vi "update devices in UI.vi"() -> ()   [LabVIEW 2025]
uses:
  <resource>/objmgr/niflexrioatomicsae.rc
panel:
  out "Ring Text.Text":string
  in  "Text Ring":u16(ring) items=["PXI1Slot2", "PXI1Slot5"]
  out "Array":string[](array[string])
  out "ProdName":string
  out "Found":bool
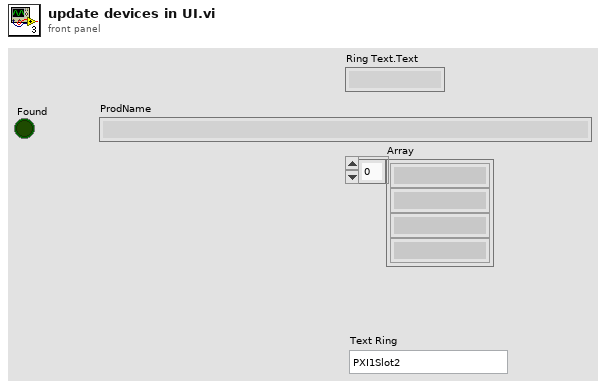
[diagram p1: front panel]
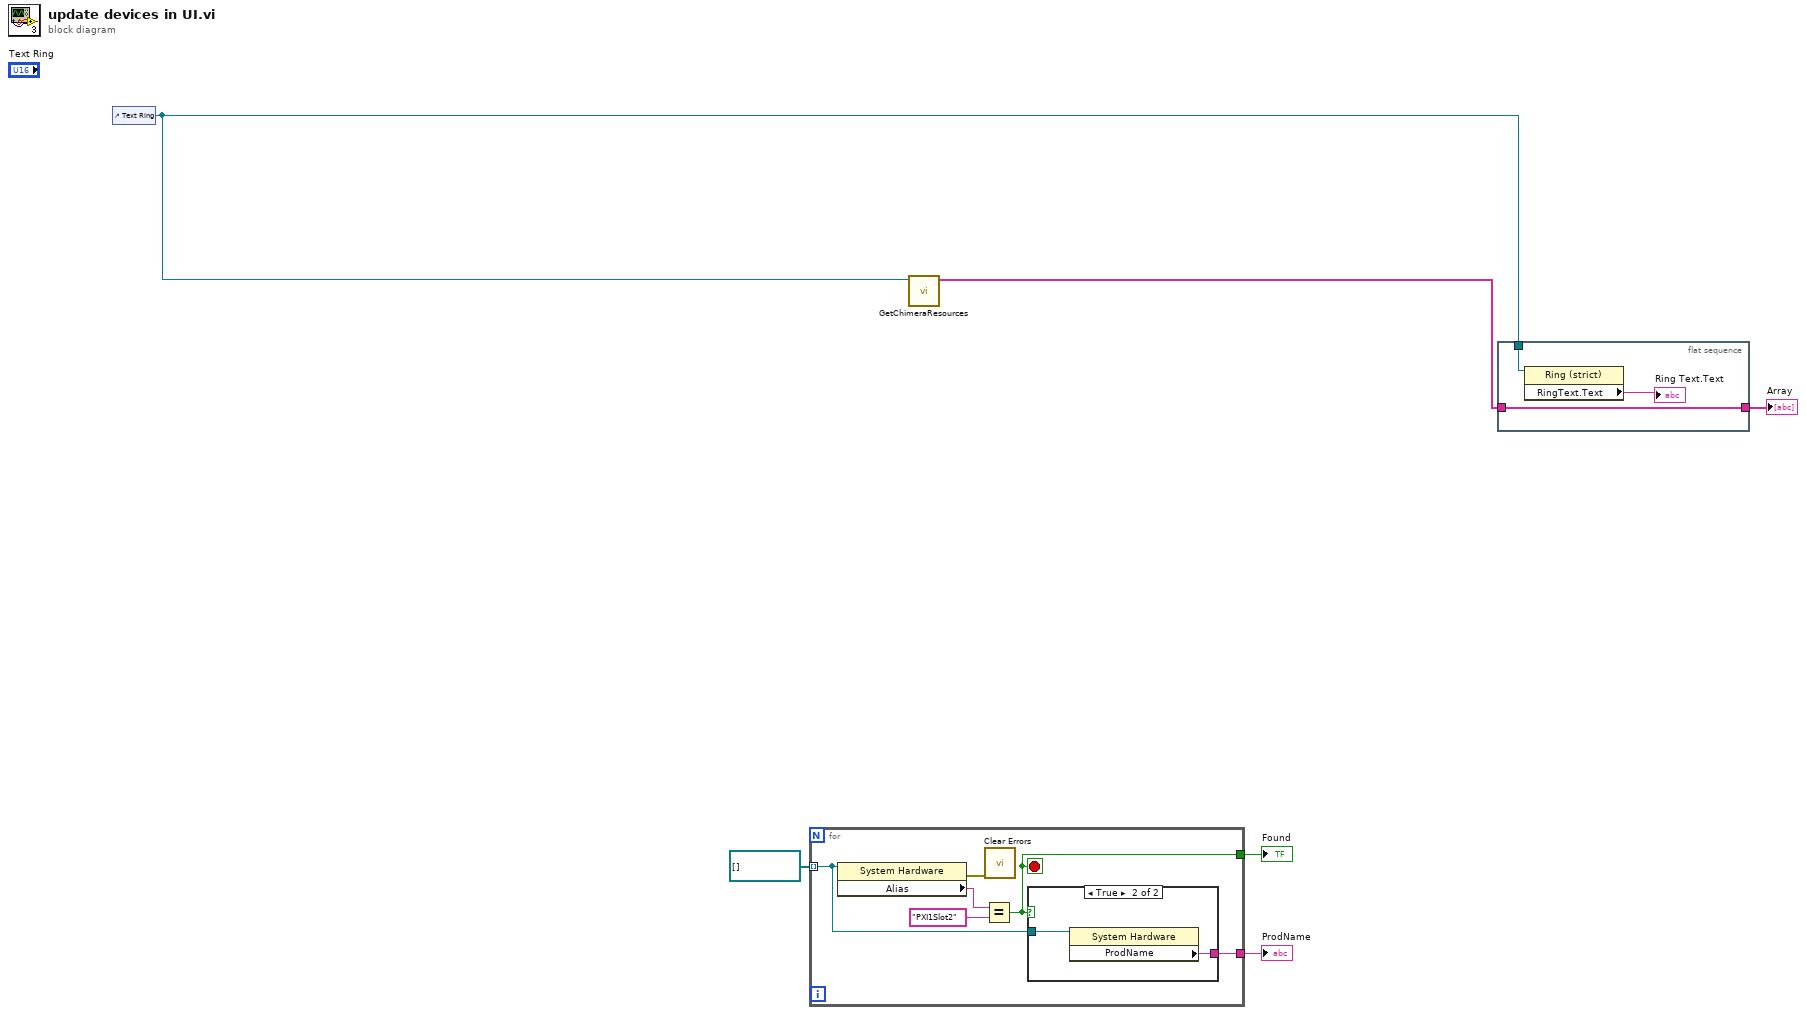
[diagram p0: block diagram]
diagram:
  n1 = control-ref of="Text Ring"() -> (w2:refnum<vi>)
  n2 = for {
    tunnel: refnum<k20>[] [] ("Resources out") -> [w10] mode=indexing
    tunnel: [w8] -> w6
    tunnel: [w9] -> w5
    stop <- w8 stop-if-true
    n3 = property class="System Hardware"(reference=w10) -> (error out=w7:errorcluster, "Alias"=w12:string)  [unwired: 1 in, 1 out]
    n4 = Equal?(x=w12, y="PXI1Slot2") -> (x = y?=w8:bool)
    n5 = call <vilib>:"Clear Errors.vi"("error in (no error)"=w7) -> ()  [unwired: 5 in, 2 out]
    n6 = case shown="True" w8 {
      tunnel: w10 -> [_ w14]
      tunnel: [_ w13] -> w9
      frame False {
      }
      frame True {
        n7 = property class="System Hardware"(reference=w14) -> ("ProdName"=w13:string)  [unwired: 1 in, 2 out]
      }
    }
  }
  "Found" <- w6
  "ProdName" <- w5
  n8 = call "GetChimeraResources.vi"("Ring in"=w2) -> ("Array"=w3:string[])  [unwired: 10 in]
  n9 = flat-sequence {
    tunnel: [w17] -> w4
    tunnel: w3 -> [w17]
    tunnel: w2 -> [w15]
    frame #0 {
      n10 = property class="Ring (strict)"(reference=w15) -> ("RingText.Text"=→"Ring Text.Text":string)  [unwired: 1 in, 2 out]
    }
  }
  "Array" <- w4
